vi "Fluence Cam Launcher.vi"() -> ()   [LabVIEW 2014, in "HIJ Vision Fluence Cam.lvlib"]
uses:
  <vilib>/userdefined/High Color/IMAQdx.ctl
  HIJ Vision Fluence Cam/HIJ Vision Fluence Cam.lvclass
  HIJ Vision Fluence Cam/HIJ Vision Fluence Cam.lvclass/HIJ Vision Fluence Cam.ctl
  Shared Code/Viewable Actor/ViewableActor Messages/Set Window Titel Msg/Set Window Titel Msg.lvclass/Set Window Titel Msg.ctl
  <vilib>/ActorFramework/Message Enqueuer/Message Enqueuer.lvclass/Message Enqueuer.ctl
  HIJ Vision Fluence Cam/Write Size of Region.vi
  HIJ Vision Fluence Cam/Write @Energy.vi
  <vilib>/ActorFramework/Message Enqueuer/Enqueue.vi
  <vilib>/Utility/config.llb/Read Key (Path).vi
  <vilib>/Utility/config.llb/Read Key (String).vi
  <vilib>/Utility/config.llb/Read Key (U32).vi
  <vilib>/Utility/config.llb/Read Key (Double).vi
  Applications/HIJ Vision Camera App/HIJ Vision Camera App/Write Start Camera.vi
  Applications/HIJ Vision Camera App/HIJ Vision Camera App/Write my ConfigDir.vi
  Applications/HIJ Vision Camera App/HIJ Vision Camera App/Write my WorkDir.vi
  <vilib>/ActorFramework/Message Priority Queue/Priority Enqueue.vi
  <vilib>/Utility/config.llb/Write Key (Path).vi
  <vilib>/Utility/config.llb/Write Key (String).vi
  <vilib>/Utility/config.llb/Write Key (U32).vi
  <vilib>/Utility/config.llb/Write Key (Double).vi
  Shared Code/Viewable Actor/ViewableActor Messages/Set Window Titel Msg/Set Window Titel Msg.lvclass
  HIJ Vision Fluence Cam.lvlib
  <vilib>/ActorFramework/Actor/Actor.lvclass
  <vilib>/Utility/config.llb/NI_LVConfig.lvlib
panel:
  out "error out":errorcluster
  in  "@Energy":dbl[unit]=10.0 format="%#_13g"
  in  "Size of Region":u8=10
  in  "Start Camera":T1="TestCam"
  in  "Start ConfigDir":path=path "C:/Users/user/Desktop/test/ConfigDir"
  in  "Start WorkDir":path=path "C:/Users/user/Desktop/test/WorkDir"
  in  "UI Cnfg":path
  in  "CLine Parameter":string
  in  "RUN_STOP":bool=TRUE
  # "px"
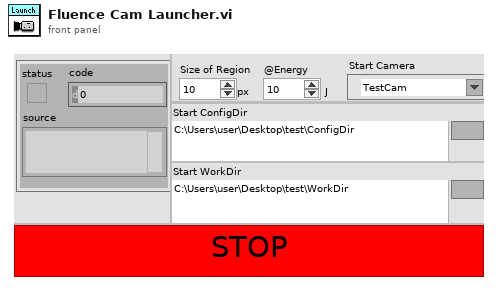
[diagram p1: front panel]
types:
  T1 = typedef "IMAQdx.ctl" = refnum<k21>
  T2 = typedef "NI_LVConfig.lvlib/Config Data RefNum.ctl" = refnum<k1>
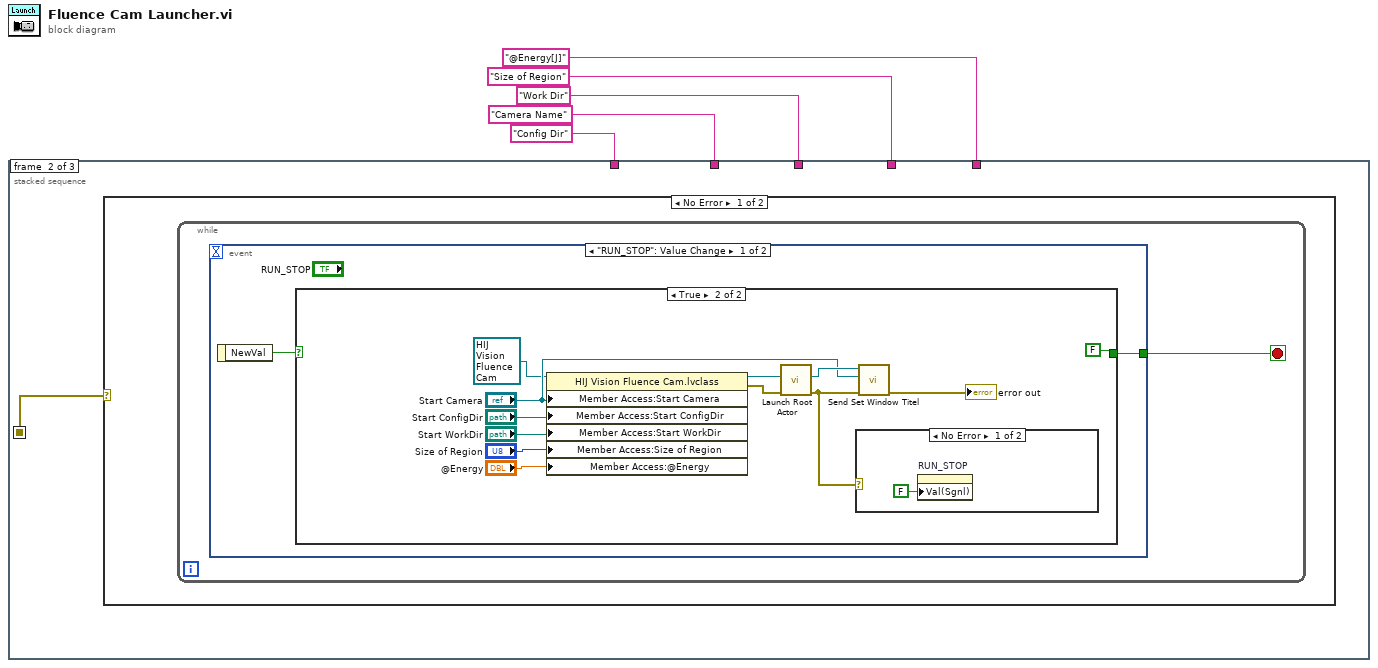
[diagram p0: block diagram]
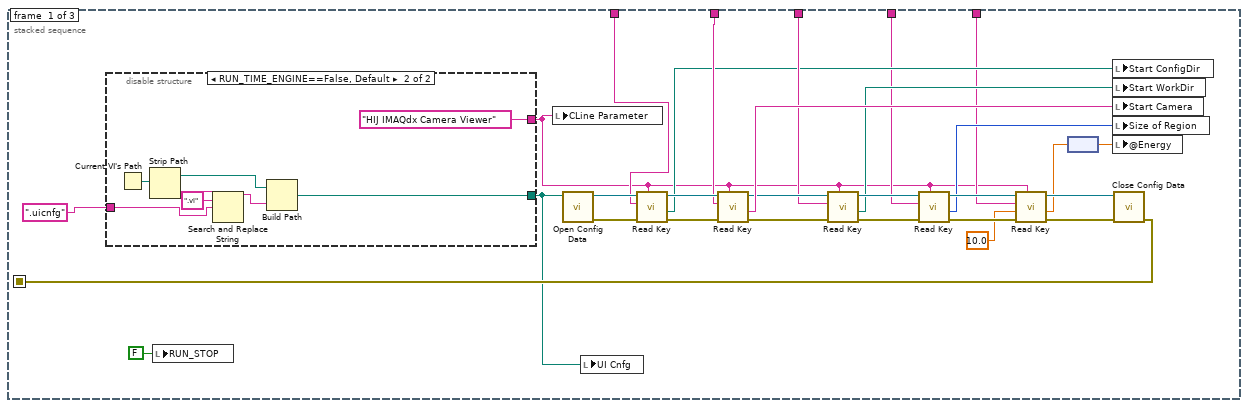
[diagram p2: hidden frame]
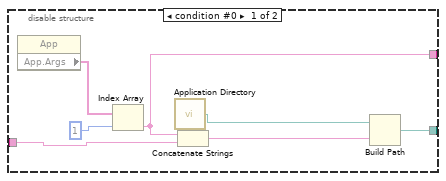
[diagram p3: hidden frame]
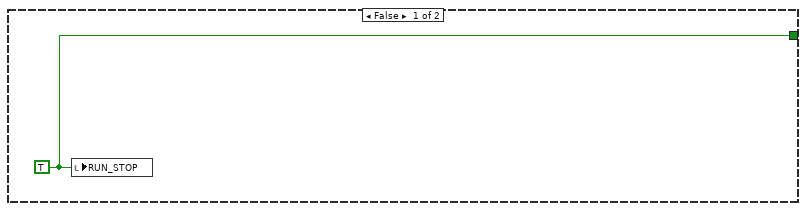
[diagram p4: hidden frame]
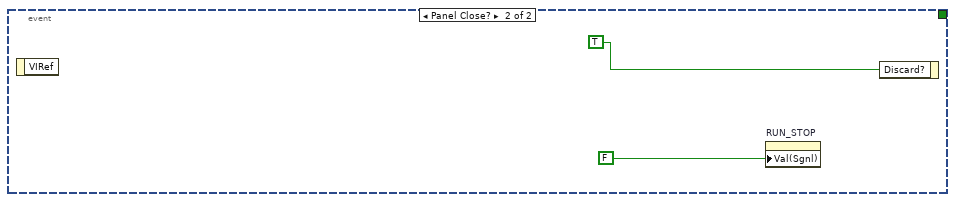
[diagram p6: hidden frame]
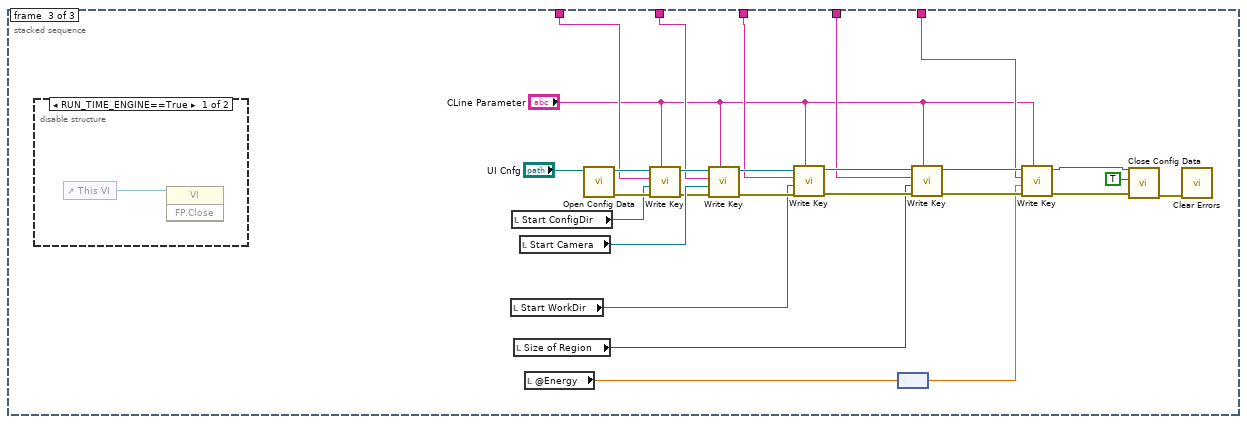
[diagram p8: hidden frame]
diagram:
  n1 = stacked-sequence {
    seq-local: [w26 _ _] -> [_ w49 _]
    tunnel: "Camera Name" ("key") -> [w28 _ w91]
    tunnel: "Config Dir" ("key") -> [w27 _ w92]
    tunnel: "Work Dir" ("key") -> [w19 _ w80]
    tunnel: "Size of Region" ("key") -> [w12 _ w77]
    tunnel: "@Energy[J]" ("key") -> [w10 _ w72]
    frame #0 {
      n2 = disable-structure shown="RUN_TIME_ENGINE==False, Default" {
        disable-tunnel: [w36 w42] -> w24
        disable-tunnel: ".uicnfg" ("string") -> [w35 w45]
        disable-tunnel: [w34 "HIJ IMAQdx Camera Viewer"] -> w9
        frame condition #0 {
          n3 = property class="App"() -> ("App.Args"=w40:string[])  [unwired: 2 in, 2 out]
          n4 = Index Array(array=w40, index=1) -> (element=w34:string)
          n5 = call <vilib>:"Application Directory.vi"() -> ("Application Directory"=w38:path)
          n6 = Concatenate Strings(w34, w35) -> (w37:string)
          n7 = Build Path(base path=w38, name or relative path=w37) -> (appended path=w36:path)
        }
        frame condition #1 (active) {
          n8 = Current VI's Path() -> (path=w48:path)
          n9 = Strip Path(path=w48) -> (stripped path=w43:path, name=w47:string)
          n10 = Search and Replace String(input string=w47, search string=".vi", replace string=w45) -> (result string=w44:string)  [unwired: 5 in, 3 out]
          n11 = Build Path(base path=w43, name or relative path=w44) -> (appended path=w42:path)
        }
      }
      n12 = local write "RUN_STOP"(FALSE ("RUN_STOP")) -> ()
      n13 = local write "CLine Parameter"(w9) -> ()
      n14 = call <vilib>:"Open Config Data.vi"("configuration file path"=w24) -> ("error out"=w30:errorcluster, "refnum"=w29:T2)  [unwired: 8 in, 1 out]
      n15 = local write "UI Cnfg"(w24) -> ()
      n16 = call-poly <vilib>:"Read Key.vi"("section"=w9, "error in (no error)"=w30, "key"=w27, "refnum"=w29) -> ("error out"=w31:errorcluster, "value"=w17:path, "refnum out"=w32:T2)  [unwired: 4 in, 1 out]
      n17 = call-poly <vilib>:"Read Key.vi"("section"=w9, "error in (no error)"=w31, "key"=w28, "refnum"=w32) -> ("error out"=w22:errorcluster, "value"=w23:string, "refnum out"=w21:T2)  [unwired: 4 in, 1 out]
      n18 = call-poly <vilib>:"Read Key.vi"("section"=w9, "error in (no error)"=w22, "key"=w19, "refnum"=w21) -> ("error out"=w14:errorcluster, "value"=w18:path, "refnum out"=w20:T2)  [unwired: 4 in, 1 out]
      n19 = call-poly <vilib>:"Read Key.vi"("section"=w9, "error in (no error)"=w14, "key"=w12, "refnum"=w20) -> ("error out"=w13:errorcluster, "value"=w15:u32, "refnum out"=w16:T2)  [unwired: 4 in, 1 out]
      n20 = call-poly <vilib>:"Read Key.vi"("section"=w9, "default value"=10.0 ("@Energy"), "key"=w10, "refnum"=w16) -> ("value"=w7:dbl, "refnum out"=w11:T2)  [unwired: 4 in, 2 out]
      n21 = node(w7) -> (w6:dbl[unit])
      n22 = local write "Start ConfigDir"(w17) -> ()
      n23 = local write "Start WorkDir"(w18) -> ()
      n24 = local write "Start Camera"(w23) -> ()
      n25 = local write "Size of Region"(w15) -> ()
      n26 = local write "@Energy"(w6) -> ()
      n27 = call <vilib>:"Close Config Data.vi"("error in (no error)"=w13, "refnum"=w11) -> ("error out"=w26:errorcluster)  [unwired: 8 in, 1 out]
    }
    frame #1 {
      n28 = case shown="No Error" w49 {
        frame No Error {
          n29 = while {
            stop <- w50 stop-if-true
            n30 = event shown="[0] \"RUN_STOP\": Value Change" {
              selector: _ -> [_ _]
              dyn-events: _ -> [_ _]
              timeout: _ -> [_ _]
              tunnel: [w52 _] -> w50
              event "RUN_STOP": Value Change {
                n31 = event-data() -> ("NewVal"=w51:bool)  [unwired: 1 in]
                n32 = case shown="True" w51 {
                  tunnel: [w53 FALSE] -> w52
                  frame False {
                    w53 = TRUE ("RUN_STOP")
                    n33 = local write "RUN_STOP"(w53) -> ()
                  }
                  frame True {
                    n34 = property class="HIJ Vision Fluence Cam.lvclass"(reference=refnum<class "HIJ Vision Fluence Cam.lvclass"> refnum ("HIJ Vision Fluence Cam.lvlib:HIJ Vision Fluence Cam.lvclass"), "Member Access:Start Camera"="Start Camera", "Member Access:Start ConfigDir"="Start ConfigDir", "Member Access:Start WorkDir"="Start WorkDir", "Member Access:Size of Region"="Size of Region", "Member Access:@Energy"="@Energy") -> (reference out=w61:refnum<class "HIJ Vision Fluence Cam.lvclass">, error out=w62:errorcluster)  [unwired: 1 in]
                    n35 = call <vilib>:"Launch Root Actor.vi"("error in (no error)"=w62, "Actor"=w61) -> ("error out"=w60:errorcluster, "Actor's Enqueuer"=w59:refnum<class "Message Enqueuer.lvclass">)  [unwired: 8 in]
                    n36 = case shown="No Error" w60 {
                      frame No Error {
                        n37 = property on="RUN_STOP" class="Bool (strict)"("Val(Sgnl)"=FALSE ("Value (Signaling)")) -> ()  [unwired: 2 in, 2 out]
                      }
                      frame Error {
                      }
                    }
                    n38 = call "Send Set Window Titel.vi"("error in (no error)"=w60, "Title"="Start Camera", "Message Enqueuer"=w59) -> ("error out"=→"error out":errorcluster)  [unwired: 7 in, 1 out]
                  }
                }
              }
              event Panel Close? {
                n39 = event-data() -> ()  [unwired: 1 in, 1 out]
                n40 = property on="RUN_STOP" class="Bool (strict)"("Val(Sgnl)"=FALSE ("Value (Signaling)")) -> ()  [unwired: 2 in, 2 out]
                n41 = event-data("Discard?"=TRUE) -> ()  [unwired: 1 in, 1 out]
              }
            }
          }
        }
        frame Error {
        }
      }
    }
    frame #2 {
      n42 = disable-structure shown="RUN_TIME_ENGINE==True" {
        frame condition #0 {
          n43 = control-ref of="This VI"() -> (w96:refnum<vi>)
          n44 = invoke class="VI" method="FP.Close"(reference=w96) -> ()  [unwired: 2 in, 3 out]
        }
        frame condition #1 (active) {
        }
      }
      n45 = local read "Start WorkDir"() -> (w81:path)
      n46 = local read "Start ConfigDir"() -> (w85:path)
      n47 = local read "Size of Region"() -> (w76:u8)
      n48 = local read "Start Camera"() -> (w90:T1)
      n49 = local read "@Energy"() -> (w70:dbl[unit])
      n50 = call <vilib>:"Open Config Data.vi"("configuration file path"="UI Cnfg") -> ("error out"=w89:errorcluster, "refnum"=w94:T2)  [unwired: 8 in, 1 out]
      n51 = call-poly <vilib>:"Write Key.vi"("section"="CLine Parameter", "error in (no error)"=w89, "value"=w85, "key"=w92, "refnum"=w94) -> ("error out"=w88:errorcluster, "refnum out"=w95:T2)  [unwired: 4 in, 1 out]
      n52 = call-poly <vilib>:"Write Key.vi"("section"="CLine Parameter", "error in (no error)"=w88, "value"=w90, "key"=w91, "refnum"=w95) -> ("error out"=w83:errorcluster, "refnum out"=w84:T2)  [unwired: 4 in, 1 out]
      n53 = call-poly <vilib>:"Write Key.vi"("section"="CLine Parameter", "error in (no error)"=w83, "value"=w81, "key"=w80, "refnum"=w84) -> ("error out"=w78:errorcluster, "refnum out"=w82:T2)  [unwired: 4 in, 1 out]
      n54 = node(w70) -> (w69:dbl)
      n55 = call-poly <vilib>:"Write Key.vi"("section"="CLine Parameter", "error in (no error)"=w78, "value"=w76, "key"=w77, "refnum"=w82) -> ("error out"=w74:errorcluster, "refnum out"=w79:T2)  [unwired: 4 in, 1 out]
      n56 = call-poly <vilib>:"Write Key.vi"("section"="CLine Parameter", "error in (no error)"=w74, "value"=w69, "key"=w72, "refnum"=w79) -> ("error out"=w73:errorcluster, "refnum out"=w75:T2)  [unwired: 4 in, 1 out]
      n57 = call <vilib>:"Close Config Data.vi"("error in (no error)"=w73, "write file if changed (T)"=TRUE, "refnum"=w75) -> ("error out"=w87:errorcluster)  [unwired: 7 in, 1 out]
      n58 = call <vilib>:"Clear Errors.vi"("error in (no error)"=w87) -> ()  [unwired: 5 in, 2 out]
    }
  }
